vi "751projectprogress.vi"() -> ()   [LabVIEW 2020]
uses:
  <vilib>/addons/control/pid/pid.llb/PID (DBL).vi
  <vilib>/addons/control/pid/NI_PID_pid.lvlib
panel:
  out "max":dbl
  in  "PID gains":T1={"proportional gain (Kc)"=1.0, "integral time (Ti, min)"=0.01, "derivative time (Td, min)"=0.0} {"derivative time (Td, min)" format="%.3f"; "integral time (Ti, min)" format="%.3f"; "proportional gain (Kc)" format="%.3f"}
  out "Measured Distance":dbl
  out "IR sensor voltage\n reading":dbl
  in  "stop":bool
  out "Proximity Sensor Voltage":dynamicdata(graph)
  out "Setpoint":dbl
  out "Unknown Resistor Value":dbl
  out "Voltage Drop":dbl
  out "Waveform Chart":dynamicdata(graph)
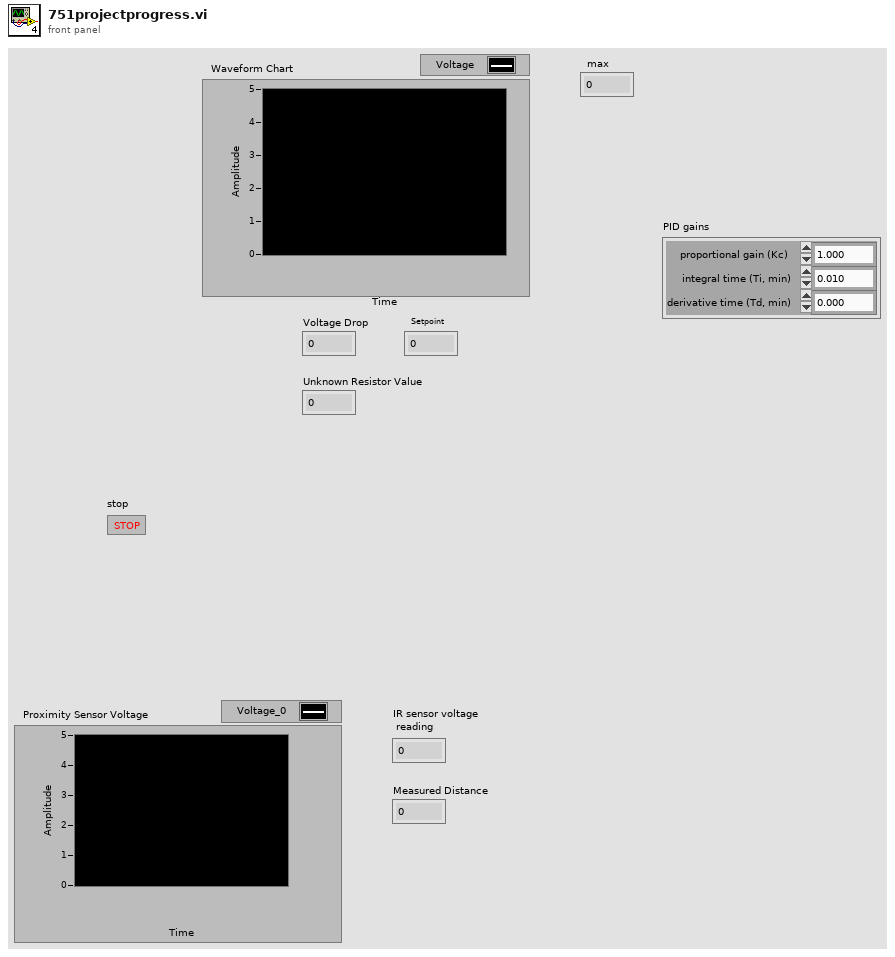
[diagram p1: front panel]
types:
  T1 = cluster{"proportional gain (Kc)":dbl, "integral time (Ti, min)":dbl, "derivative time (Td, min)":dbl}
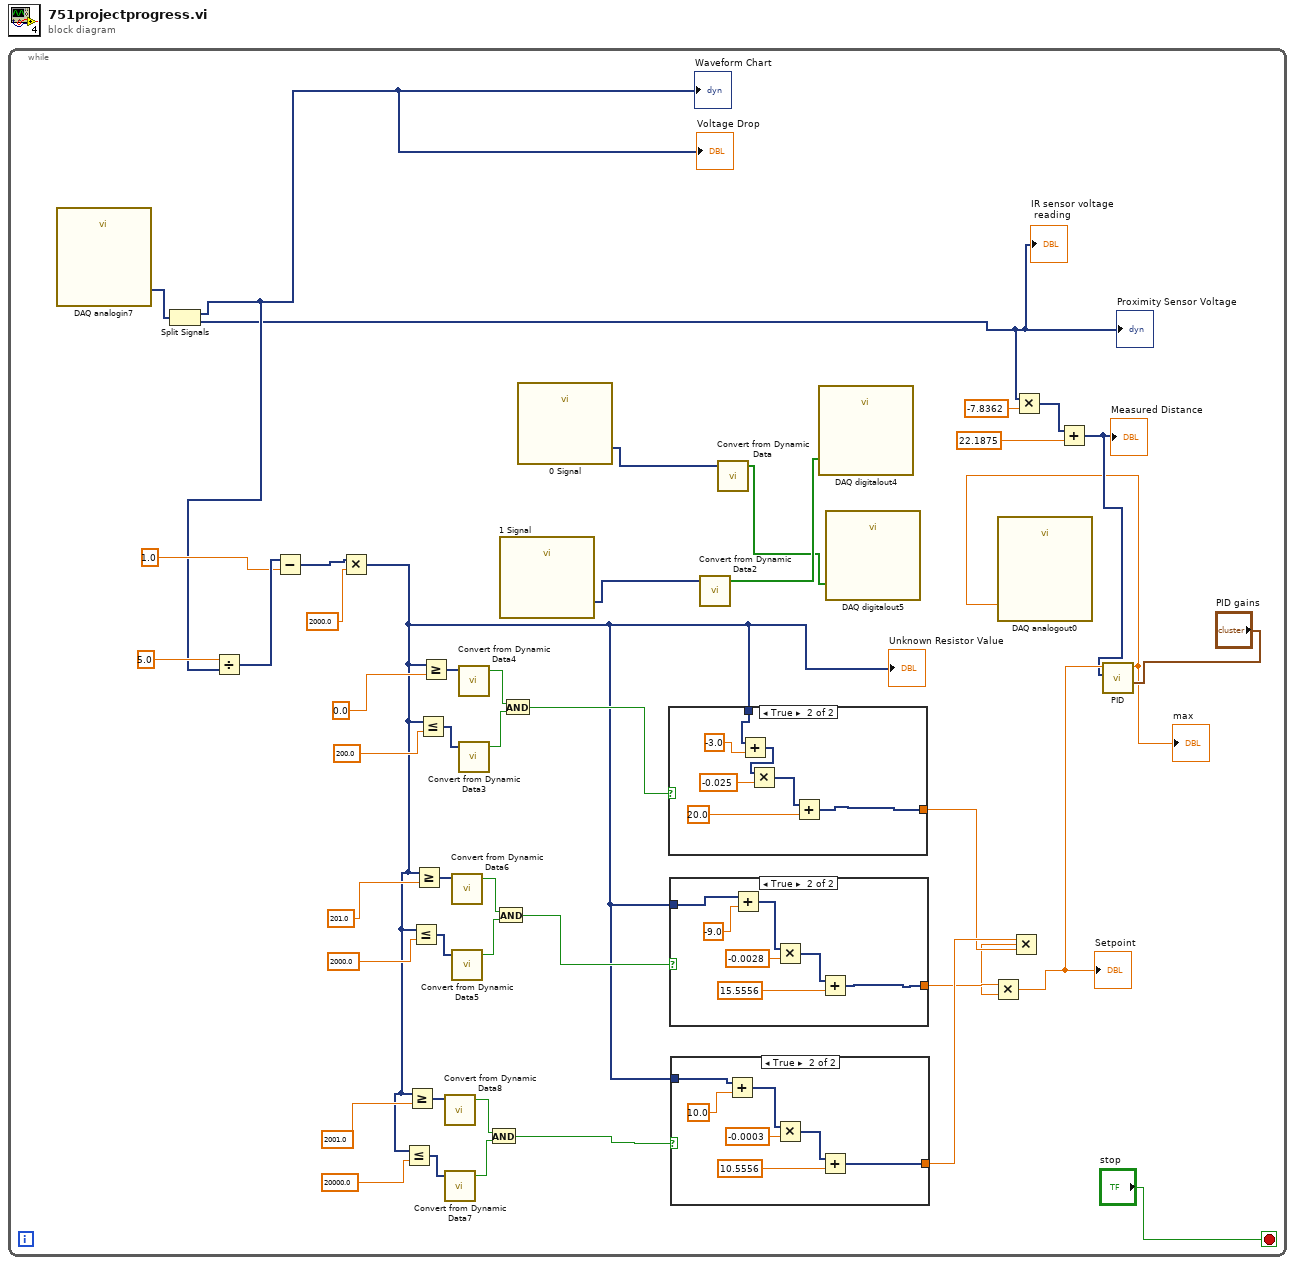
[diagram p0: block diagram]
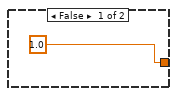
[diagram p2: hidden frame]
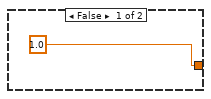
[diagram p3: hidden frame]
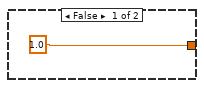
[diagram p4: hidden frame]
diagram:
  n1 = while {
    stop <- "stop" stop-if-true
    n2 = call "DAQ analogin7"() -> ("data"=w10:dynamicdata)  [unwired: 17 in, 2 out]
    n3 = Split Signals(w10) -> (w11:dynamicdata, w5:dynamicdata)  [unwired: 2 in]
    "Waveform Chart" <- w11
    "Voltage Drop" <- w11
    "Proximity Sensor Voltage" <- w5
    "IR sensor voltage\n reading" <- w5
    n4 = Divide(x=5.0, y=w11) -> (x/y=w21:dynamicdata)
    n5 = Subtract(x=w21, y=1.0) -> (x-y=w22:dynamicdata)
    n6 = Multiply(x=w22, y=2000.0) -> (x*y=w16:dynamicdata)
    "Unknown Resistor Value" <- w16
    n7 = Less Or Equal?(x=w16, y=20000.0) -> (x <= y?=w26:dynamicdata)
    n8 = Greater Or Equal?(x=w16, y=2001.0) -> (x >= y?=w24:dynamicdata)
    n9 = Less Or Equal?(x=w16, y=2000.0) -> (x <= y?=w32:dynamicdata)
    n10 = Greater Or Equal?(x=w16, y=201.0) -> (x >= y?=w30:dynamicdata)
    n11 = Less Or Equal?(x=w16, y=200.0) -> (x <= y?=w38:dynamicdata)
    n12 = Greater Or Equal?(x=w16, y=0.0) -> (x >= y?=w36:dynamicdata)
    n13 = call "Convert from Dynamic Data8"("Dynamic Data Type"=w24) -> ("Scalar"=w23:bool)  [unwired: 3 in]
    n14 = call "Convert from Dynamic Data7"("Dynamic Data Type"=w26) -> ("Scalar"=w25:bool)  [unwired: 3 in]
    n15 = call "Convert from Dynamic Data6"("Dynamic Data Type"=w30) -> ("Scalar"=w29:bool)  [unwired: 3 in]
    n16 = call "Convert from Dynamic Data5"("Dynamic Data Type"=w32) -> ("Scalar"=w31:bool)  [unwired: 3 in]
    n17 = call "Convert from Dynamic Data4"("Dynamic Data Type"=w36) -> ("Scalar"=w35:bool)  [unwired: 3 in]
    n18 = call "Convert from Dynamic Data3"("Dynamic Data Type"=w38) -> ("Scalar"=w37:bool)  [unwired: 3 in]
    n19 = And(x=w23, y=w25) -> (x .and. y?=w19:bool)
    n20 = And(x=w29, y=w31) -> (x .and. y?=w18:bool)
    n21 = call "1 Signal"() -> ("DC"=w45:dynamicdata)  [unwired: 14 in, 1 out]
    n22 = And(x=w35, y=w37) -> (x .and. y?=w17:bool)
    n23 = call "0 Signal"() -> ("DC"=w46:dynamicdata)  [unwired: 14 in, 1 out]
    n24 = case shown="True" w17 {
      tunnel: w16 -> [_ w65]
      tunnel: [1.0 w67] -> w14
      frame False {
      }
      frame True {
        n25 = Add(x=w65, y=-3.0) -> (x+y=w66:dynamicdata)
        n26 = Multiply(x=w66, y=-0.025) -> (x*y=w68:dynamicdata)
        n27 = Add(x=w68, y=20.0) -> (x+y=w67:dynamicdata)
      }
    }
    n28 = case shown="True" w18 {
      tunnel: w16 -> [_ w57]
      tunnel: [1.0 w59] -> w13
      frame False {
      }
      frame True {
        n29 = Add(x=w57, y=-9.0) -> (x+y=w56:dynamicdata)
        n30 = Multiply(x=w56, y=-0.0028) -> (x*y=w60:dynamicdata)
        n31 = Add(x=w60, y=15.5556) -> (x+y=w59:dynamicdata)
      }
    }
    n32 = case shown="True" w19 {
      tunnel: w16 -> [_ w49]
      tunnel: [1.0 w51] -> w15
      frame False {
      }
      frame True {
        n33 = Add(x=w49, y=10.0) -> (x+y=w50:dynamicdata)
        n34 = Multiply(x=w50, y=-0.0003) -> (x*y=w52:dynamicdata)
        n35 = Add(x=w52, y=10.5556) -> (x+y=w51:dynamicdata)
      }
    }
    n36 = call "Convert from Dynamic Data2"("Dynamic Data Type"=w45) -> ("Array"=w44:bool[])  [unwired: 3 in]
    n37 = call "Convert from Dynamic Data"("Dynamic Data Type"=w46) -> ("Array"=w43:bool[])  [unwired: 3 in]
    n38 = call "DAQ digitalout4"("data"=w44) -> ()  [unwired: 17 in, 2 out]
    n39 = call "DAQ digitalout5"("data"=w43) -> ()  [unwired: 17 in, 2 out]
    n40 = Multiply(x=w15, y=w14) -> (x*y=w12:dbl)
    n41 = Multiply(x=w13, y=w12) -> (x*y=w3:dbl)
    "Setpoint" <- w3
    n42 = Multiply(x=w5, y=-7.8362) -> (x*y=w6:dynamicdata)
    n43 = Add(x=w6, y=22.1875) -> (x+y=w2:dynamicdata)
    "Measured Distance" <- w2
    n44 = call-poly <vilib>:"PID.vi"("PID gains"="PID gains", "process variable"=w2, "setpoint"=w3) -> ("output"=w1:dbl)  [unwired: 7 in, 1 out]
    "max" <- w1
    n45 = call "DAQ analogout0"("data"=w1) -> ()  [unwired: 17 in, 2 out]
  }
